vi "Move Stage.vi"(8 "error in (no error)":errorcluster, 9 "Y Axis":dbl, 10 "X Axis":dbl, 11 "2-Axis Stage in":refnum<class "XY Stage Controller.lvclass">) -> (0 "error out":errorcluster, 3 "2-Axis Stage out":refnum<class "XY Stage Controller.lvclass">)   [LabVIEW 2022 SP3, in "XY Stage Controller.lvclass"]
uses:
  XY Stage Controller.lvclass
  XY Stage Controller.lvclass/XY Stage Controller.ctl
  XY Stage Process/XY Stage Process/XY Stage Process Messages/Move Stage Msg/Move Stage Msg.lvclass
  XY Stage Data Class/XY Stage Data Class.lvclass
  <vilib>/ErrorRing/Error Ring.xnode
  <vilib>/Utility/error.llb/Error Cluster From Error Code.vi
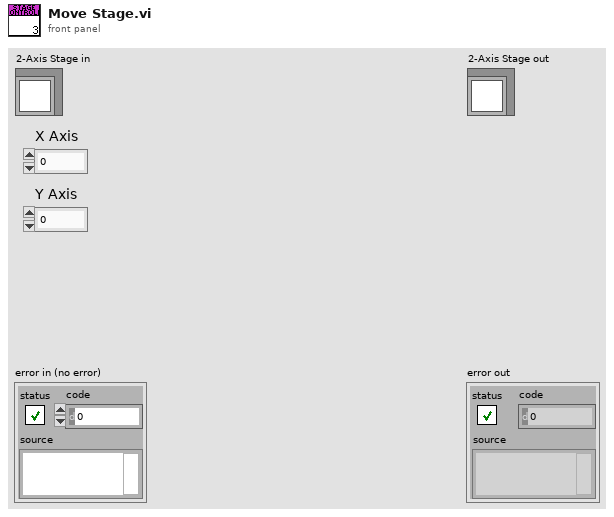
[diagram p1: front panel]
types:
  T1 = typedef "XY Stage Data Class.lvclass/Homed.ctl" = cluster{"X Homed":bool, "Y Homed":bool}
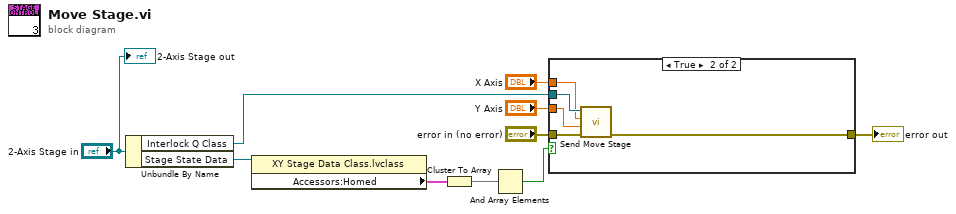
[diagram p0: block diagram]
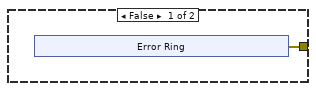
[diagram p2: hidden frame]
diagram:
  n1 = Unbundle By Name("2-Axis Stage in") -> ("Interlock Q Class"=w9:refnum<class "Interlock Q Class.lvclass">, "Stage State Data"=w4:refnum<data-value>)
  n2 = property class="XY Stage Data Class.lvclass"(reference=w4) -> ("Accessors:Homed"=w3:T1)  [unwired: 1 in, 2 out]
  n3 = Cluster To Array(cluster=w3) -> (array=w2:bool[])
  n4 = And Array Elements(Boolean array=w2) -> (logical AND=w1:bool)
  n5 = case shown="True" w1 {
    tunnel: w9 -> [_ w21]
    tunnel: "X Axis" -> [_ w20]
    tunnel: "Y Axis" -> [_ w19]
    tunnel: "error in (no error)" -> [_ w18]
    tunnel: [w11 w17] -> w5
    frame False {
      n6 = xnode "Error Ring"() -> ("error out"=w11:errorcluster)
    }
    frame True {
      n7 = call "Send Move Stage.vi"("error in (no error)"=w18, "Y Axis"=w19, "X Axis"=w20, "Interlock Q Class"=w21) -> ("error out"=w17:errorcluster)  [unwired: 6 in, 1 out]
    }
  }
  "error out" <- w5
  "2-Axis Stage out" <- "2-Axis Stage in"
